vi "getAll.vi"(8 "error in (no error)":errorcluster, 11 "Instrument.VoltageSource in":refnum<class "Instrument.VoltageSource.lvclass">) -> (0 "error out":errorcluster, 2 "getAll":variant, 3 "Instrument.VoltageSource out":refnum<class "Instrument.VoltageSource.lvclass">)   [LabVIEW 2016, in "Instrument.VoltageSource.lvclass"]
uses:
  Instrument.VoltageSource.lvclass
  Typedefs/getAll.ctl
  Instrument.VoltageSource.lvclass/Instrument.VoltageSource.ctl
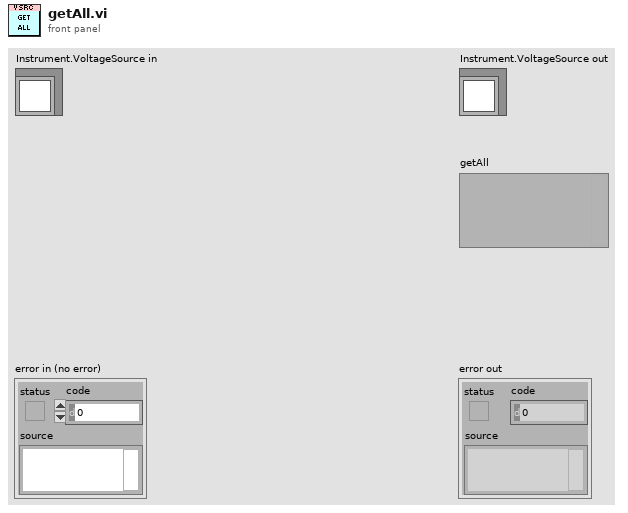
[diagram p1: front panel]
types:
  T1 = typedef "Instrument.VoltageSource.lvclass/getAll.ctl" = cluster{"Amplified Output":dbl, "DAQ Output":dbl, "Amplifier Gain":dbl}
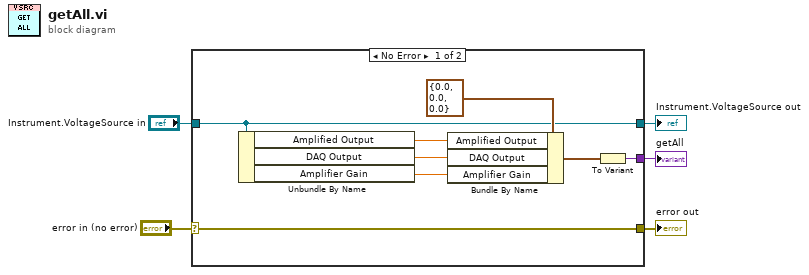
[diagram p0: block diagram]
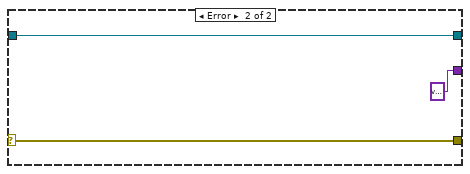
[diagram p2: hidden frame]
diagram:
  n1 = case shown="No Error" "error in (no error)" {
    selector: "error in (no error)" -> [w7 w16]
    tunnel: [w8 variant ("Variant")] -> w5
    tunnel: "Instrument.VoltageSource in" -> [w6 w15]
    tunnel: [w7 w16] -> w2
    tunnel: [w6 w15] -> w1
    frame No Error {
      n2 = Unbundle By Name(w6) -> ("Amplified Output"=w11:dbl, "DAQ Output"=w10:dbl, "Amplifier Gain"=w12:dbl)
      n3 = Bundle By Name(cluster=T1 {"Amplified Output"=0.0, "DAQ Output"=0.0, "Amplifier Gain"=0.0}, "Amplified Output"=w11, "DAQ Output"=w10, "Amplifier Gain"=w12) -> (w9:T1)
      n4 = To Variant(anything=w9) -> (Variant=w8:variant)
    }
    frame Error {
    }
  }
  "error out" <- w2
  "Instrument.VoltageSource out" <- w1
  "getAll" <- w5
